vi "Read Module Menu Name.vi"(8 "error in":errorcluster, 11 "System Diagnostics editor node in":refnum<class "System Diagnostics editor node.lvclass">) -> (0 "error out":errorcluster, 2 "Menu Name":string, 3 "System Diagnostics editor node out":refnum<class "System Diagnostics editor node.lvclass">)   [LabVIEW 2013, in "System Diagnostics editor node.lvclass"]
uses:
  System Diagnostics editor node.lvclass
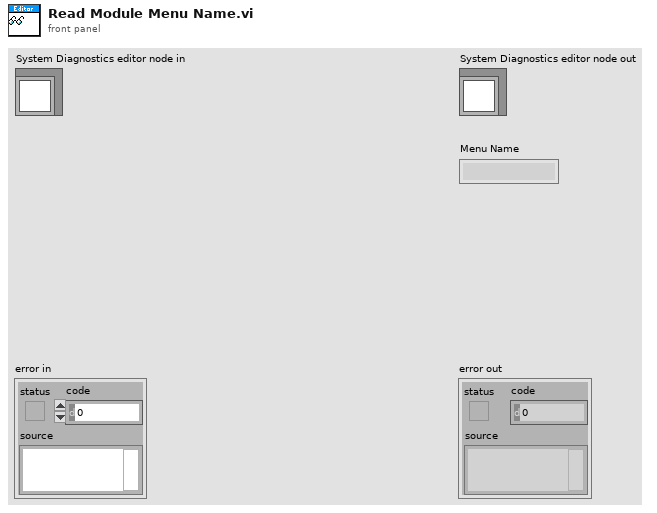
[diagram p1: front panel]
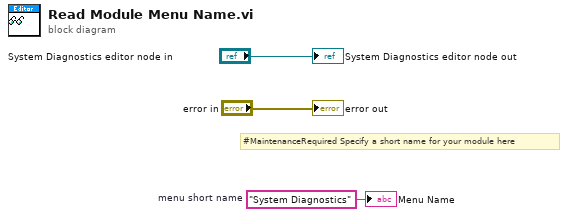
[diagram p0: block diagram]
diagram:
  w1 = "System Diagnostics"  # menu short name
  # "#MaintenanceRequired Specify a short name for your module here"
  "error out" <- "error in"
  "System Diagnostics editor node out" <- "System Diagnostics editor node in"
  "Menu Name" <- w1
